vi "MeasureParameters_to_byte.vi"(8 "error in (no error)":errorcluster, 10 "MeasConfigType":T1, 11 "UV-VIS_AVANTES in":refnum<class "UV-VIS_AVANTES.lvclass">) -> (0 "error out":errorcluster, 2 "Measure byte  array":u8[](array[numeric]), 3 "UV-VIS_AVANTES out":refnum<class "UV-VIS_AVANTES.lvclass">)   [LabVIEW 2015, in "UV-VIS_AVANTES.lvclass"]
uses:
  UV-VIS_AVANTES.lvclass
  def_measure_parameters.ctl
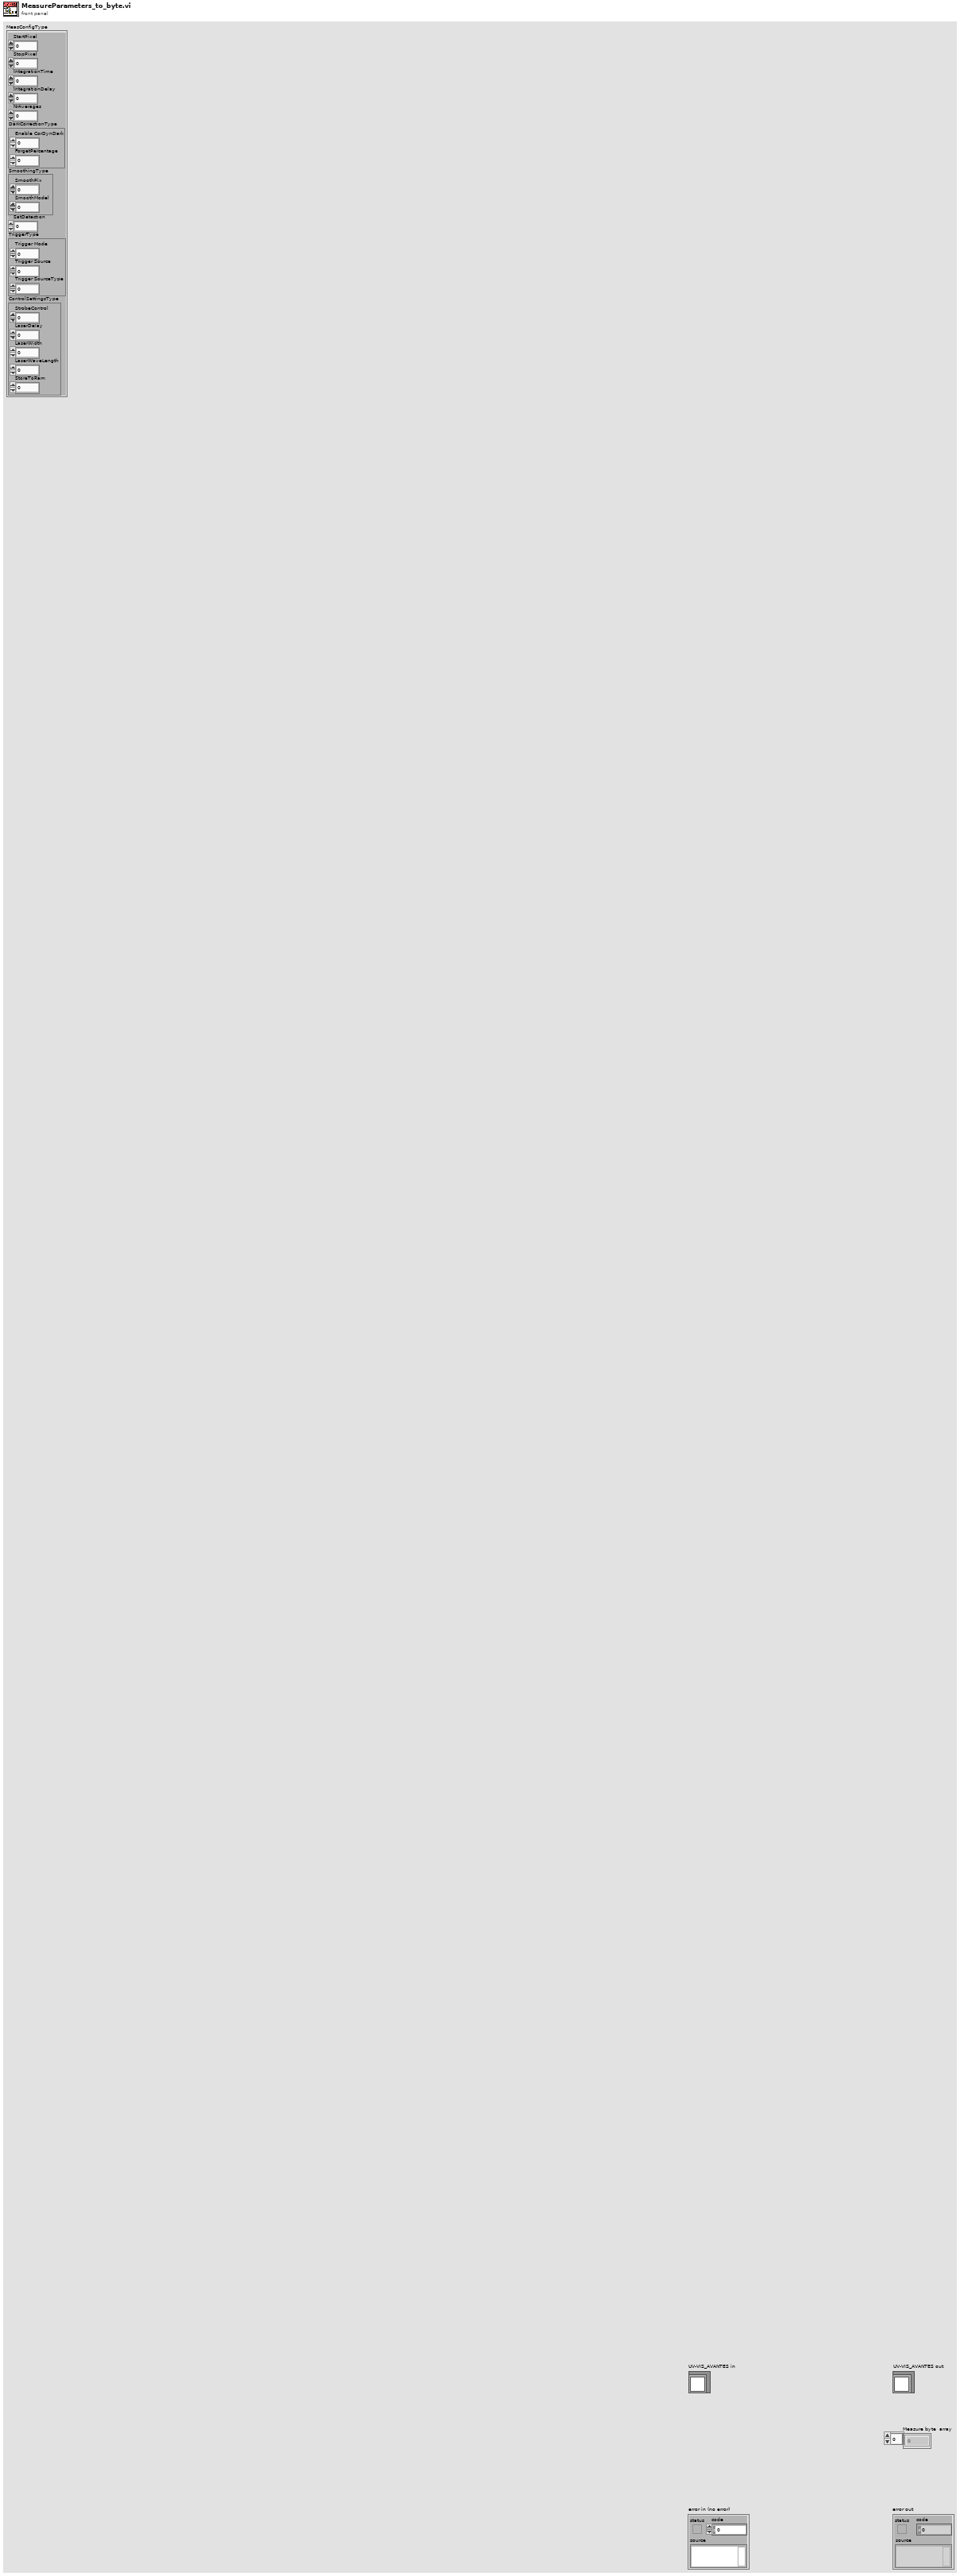
[diagram p1: front panel]
types:
  T1 = typedef "def_measure_parameters.ctl" = cluster{"StartPixel":u16, "StopPixel":u16, "IntegrationTime":sgl, "IntegrationDelay":u32, "NrAverages":u32, "DarkCorrectionType":cluster{"Enable CorDynDark":u8, "ForgetPercentage":u8}, "SmoothingType":cluster{"SmoothPix":u16, "SmoothModel":u8}, "SatDetection":u8, "TriggerType":cluster{"Trigger Mode":u8, "Trigger Source":u8, "Trigger SourceType":u8}, "ControlSettingsType":cluster{"StrobeControl":u16, "LaserDelay":u32, "LaserWidth":u32, "LaserWaveLength":sgl, "StoreToRam":u16}}
  T2 = cluster{"Enable CorDynDark":u8, "ForgetPercentage":u8}
  T3 = cluster{"Trigger Mode":u8, "Trigger Source":u8, "Trigger SourceType":u8}
  T4 = cluster{"StrobeControl":u16, "LaserDelay":u32, "LaserWidth":u32, "LaserWaveLength":sgl, "StoreToRam":u16}
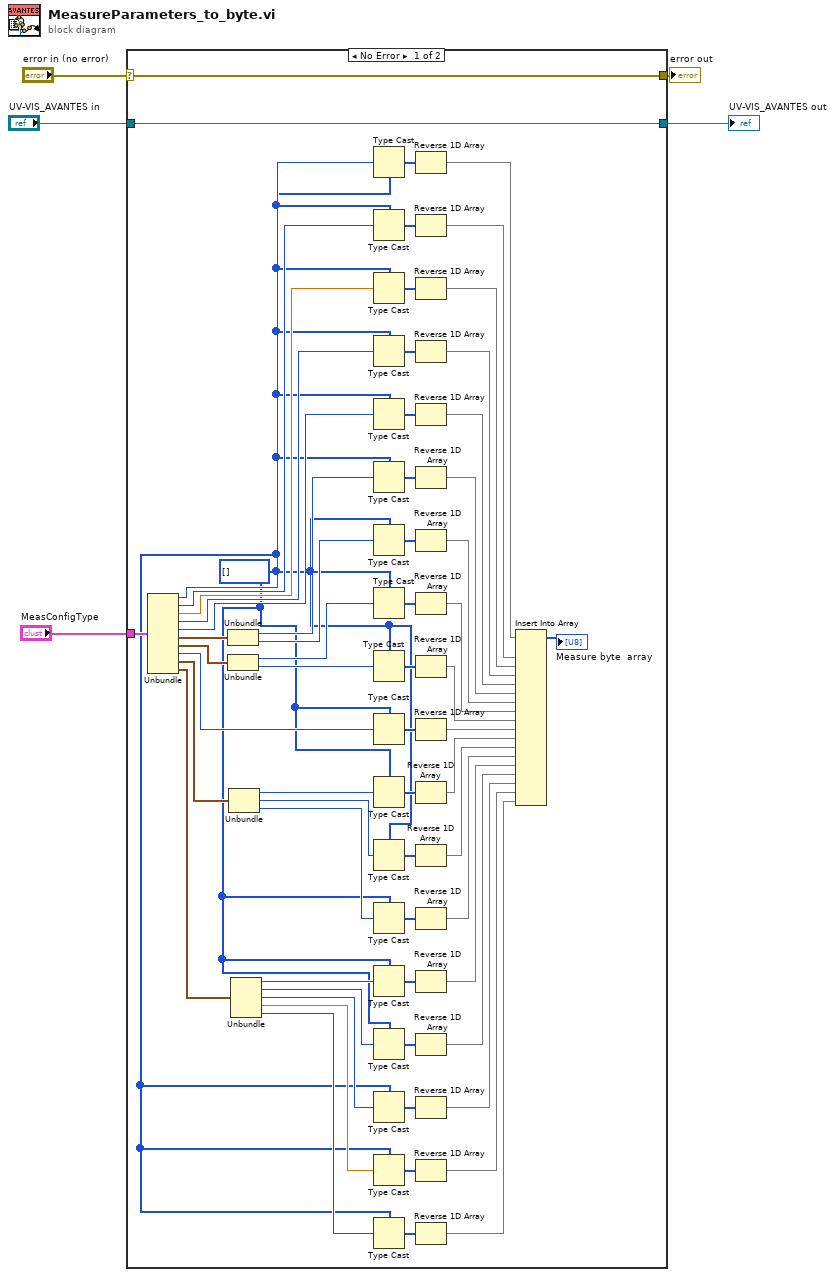
[diagram p0: block diagram]
diagram:
  n1 = case shown="No Error" "error in (no error)" {
    selector: "error in (no error)" -> [w68 w70]
    tunnel: "UV-VIS_AVANTES in" -> [w7 w69]
    tunnel: [w68 w70] -> w3
    tunnel: [w7 w69] -> w2
    tunnel: "MeasConfigType" -> [w9 _]
    frame No Error {
      w8 = u8[] [] ("ByteArray")
      n2 = Unbundle(w9) -> ("StartPixel"=w19:u16, "StopPixel"=w20:u16, "IntegrationTime"=w21:sgl, "IntegrationDelay"=w22:u32, "NrAverages"=w23:u32, "DarkCorrectionType"=w10:T2, "SmoothingType"=w11:cluster{"SmoothPix":u16, "SmoothModel":u8}, "SatDetection"=w33:u8, "TriggerType"=w12:T3, "ControlSettingsType"=w13:T4)
      n3 = Unbundle(w10) -> ("Enable CorDynDark"=w29:u8, "ForgetPercentage"=w30:u8)
      n4 = Unbundle(w11) -> ("SmoothPix"=w31:u16, "SmoothModel"=w32:u8)
      n5 = Unbundle(w12) -> ("Trigger Mode"=w51:u8, "Trigger Source"=w52:u8, "Trigger SourceType"=w53:u8)
      n6 = Unbundle(w13) -> ("StrobeControl"=w54:u16, "LaserDelay"=w55:u32, "LaserWidth"=w56:u32, "LaserWaveLength"=w57:sgl, "StoreToRam"=w58:u16)
      n7 = Type Cast(type=w8, x=w19) -> (*(type *) &x=w18:u8[])
      n8 = Type Cast(type=w8, x=w20) -> (*(type *) &x=w17:u8[])
      n9 = Type Cast(type=w8, x=w21) -> (*(type *) &x=w16:u8[])
      n10 = Type Cast(type=w8, x=w22) -> (*(type *) &x=w15:u8[])
      n11 = Type Cast(type=w8, x=w23) -> (*(type *) &x=w14:u8[])
      n12 = Type Cast(type=w8, x=w29) -> (*(type *) &x=w24:u8[])
      n13 = Type Cast(type=w8, x=w30) -> (*(type *) &x=w25:u8[])
      n14 = Type Cast(type=w8, x=w31) -> (*(type *) &x=w26:u8[])
      n15 = Type Cast(type=w8, x=w32) -> (*(type *) &x=w27:u8[])
      n16 = Type Cast(type=w8, x=w33) -> (*(type *) &x=w28:u8[])
      n17 = Type Cast(type=w8, x=w51) -> (*(type *) &x=w48:u8[])
      n18 = Type Cast(type=w8, x=w52) -> (*(type *) &x=w49:u8[])
      n19 = Type Cast(type=w8, x=w53) -> (*(type *) &x=w50:u8[])
      n20 = Type Cast(type=w8, x=w54) -> (*(type *) &x=w47:u8[])
      n21 = Type Cast(type=w8, x=w55) -> (*(type *) &x=w46:u8[])
      n22 = Type Cast(type=w8, x=w56) -> (*(type *) &x=w45:u8[])
      n23 = Type Cast(type=w8, x=w57) -> (*(type *) &x=w44:u8[])
      n24 = Type Cast(type=w8, x=w58) -> (*(type *) &x=w43:u8[])
      n25 = Reverse 1D Array(array=w18) -> (reversed array=w67:u8[])
      n26 = Reverse 1D Array(array=w17) -> (reversed array=w34:u8[])
      n27 = Reverse 1D Array(array=w16) -> (reversed array=w35:u8[])
      n28 = Reverse 1D Array(array=w15) -> (reversed array=w36:u8[])
      n29 = Reverse 1D Array(array=w14) -> (reversed array=w37:u8[])
      n30 = Reverse 1D Array(array=w24) -> (reversed array=w38:u8[])
      n31 = Reverse 1D Array(array=w25) -> (reversed array=w39:u8[])
      n32 = Reverse 1D Array(array=w26) -> (reversed array=w40:u8[])
      n33 = Reverse 1D Array(array=w27) -> (reversed array=w41:u8[])
      n34 = Reverse 1D Array(array=w28) -> (reversed array=w42:u8[])
      n35 = Reverse 1D Array(array=w48) -> (reversed array=w59:u8[])
      n36 = Reverse 1D Array(array=w49) -> (reversed array=w60:u8[])
      n37 = Reverse 1D Array(array=w50) -> (reversed array=w61:u8[])
      n38 = Reverse 1D Array(array=w47) -> (reversed array=w62:u8[])
      n39 = Reverse 1D Array(array=w46) -> (reversed array=w63:u8[])
      n40 = Reverse 1D Array(array=w45) -> (reversed array=w64:u8[])
      n41 = Reverse 1D Array(array=w44) -> (reversed array=w65:u8[])
      n42 = Reverse 1D Array(array=w43) -> (reversed array=w66:u8[])
      n43 = Insert Into Array(array=w67, new element #1=w34, new element #2=w35, new element #3=w36, new element #4=w37, new element #5=w38, new element #6=w39, new element #7=w40, new element #8=w41, new element #9=w42, new element #10=w59, new element #11=w60, new element #12=w61, new element #13=w62, new element #14=w63, new element #15=w64, new element #16=w65, new element #17=w66) -> (→"Measure byte  array":u8[])  [unwired: 1 in]
    }
    frame Error {
    }
  }
  "error out" <- w3
  "UV-VIS_AVANTES out" <- w2
